vi "Get Category.vi"(8 "error in (no error)":errorcluster, 11 "TDMS datalogger editor node in":refnum<class "TDMS datalogger editor node.lvclass">) -> (0 "error out":errorcluster, 2 "Category":string, 3 "TDMS datalogger editor node out":refnum<class "TDMS datalogger editor node.lvclass">)   [LabVIEW 2015, in "TDMS datalogger editor node.lvclass"]
uses:
  TDMS datalogger editor node.lvclass
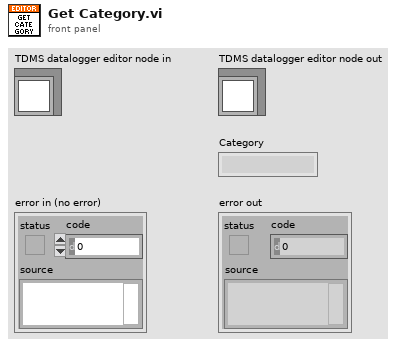
[diagram p1: front panel]
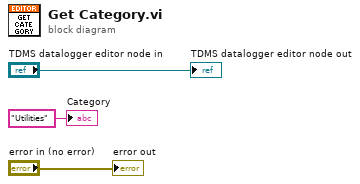
[diagram p0: block diagram]
diagram:
  "error out" <- "error in (no error)"
  "TDMS datalogger editor node out" <- "TDMS datalogger editor node in"
  "Category" <- "Utilities" ("Category")
